vi "Set Trigger Level (SubVI).vi"(2 "error in":errorcluster, 3 "Trigger Level (% of Scale)":dbl=10.0 min=0.1 max=99.9 step=0.1 format="%_3f", 4 "VISA Refnum in":refnum<visa-resource-name>) -> (0 "error out":errorcluster, 1 "VISA Refnum out":refnum<visa-resource-name>)   [LabVIEW 2017]
doc: "Set Multiplier.\nU-Link only accept 2 digit. Check and cut the number if necessary.\nWrite the data on the COM port and check if a message is sent (to control carriage data). \nMade by Tanguy BOULARD\nTHALES FRANCE"
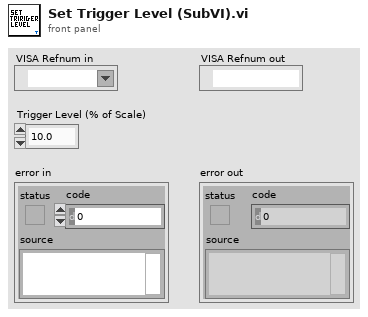
[diagram p1: front panel]
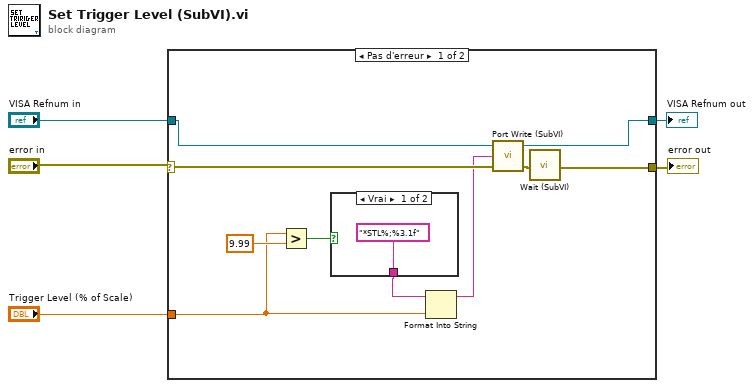
[diagram p0: block diagram]
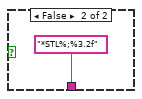
[diagram p2: hidden frame]
diagram:
  n1 = case shown="Pas d'erreur" "error in" {
    selector: "error in" -> [w15 w19]
    tunnel: [w9 w19] -> w4
    tunnel: "Trigger Level (% of Scale)" -> [w11 _]
    tunnel: "VISA Refnum in" -> [w7 w18]
    tunnel: [w8 w18] -> w1
    frame No Error {
      n2 = Greater?(x=w11, y=9.99) -> (0:w12:bool)
      n3 = case shown="Vrai" w12 {
        tunnel: ["*STL%;%3.1f" ("format string") "*STL%;%3.2f" ("format string")] -> w14
        frame True {
        }
        frame False {
        }
      }
      n4 = Format Into String(format string=w14, w11) -> (resulting string=w6:string)  [unwired: 2 in, 1 out]
      n5 = call "Port Write (SubVI).vi"("error in"=w15, "write buffer"=w6, "VISA Refnum in"=w7) -> ("error out"=w10:errorcluster, "VISA Refnum out"=w8:refnum<visa-resource-name>)  [unwired: 1 in]
      n6 = call "Wait (SubVI).vi"("error in"=w10) -> ("error out"=w9:errorcluster)  [unwired: 26 in]
    }
    frame Error {
    }
  }
  "error out" <- w4
  "VISA Refnum out" <- w1
